vi "Array Max & Min JSON.vi"(7 "JSON Array":refnum<class "JSON Array.lvclass">, 11 "error in (no error)":errorcluster) -> (4 "max value":refnum<class "JSON Null.lvclass">, 6 "max index":i32, 8 "min value":refnum<class "JSON Null.lvclass">, 10 "min index":i32, 15 "error out":errorcluster)   [LabVIEW 2015, in "LVJSON.lvlib" / "JSON Array.lvclass"]
doc: "Finds the maximum value and minimum value of the elements in a JSON Array. The elements must all be the same literal type."
uses:
  JSON Array.lvclass
  JSON Datatype/JSON Null.lvclass
  JSON String/Read value (String).vi
  JSON Helper/To More Specific Type (String).vi
  JSON Numeric/Read value (Numeric).vi
  JSON Helper/To More Specific Type (Numeric).vi
  JSON Helper/JSON Helper.lvclass
  JSON Basic Type/JSON Literal.lvclass
  JSON Numeric/JSON Numeric.lvclass
  JSON String/JSON String.lvclass
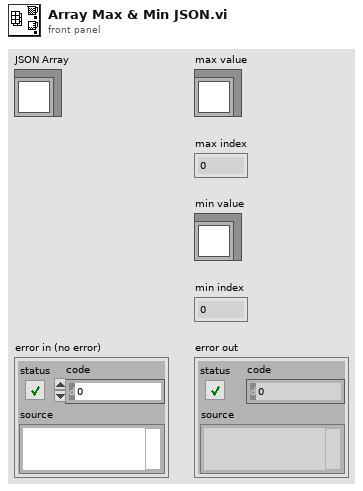
[diagram p1: front panel]
types:
  T1 = typedef "LVJSON.lvlib/JSON Types.ctl" = enum16{"String", "Numeric", "Boolean", "NULL", "Object", "Array"}
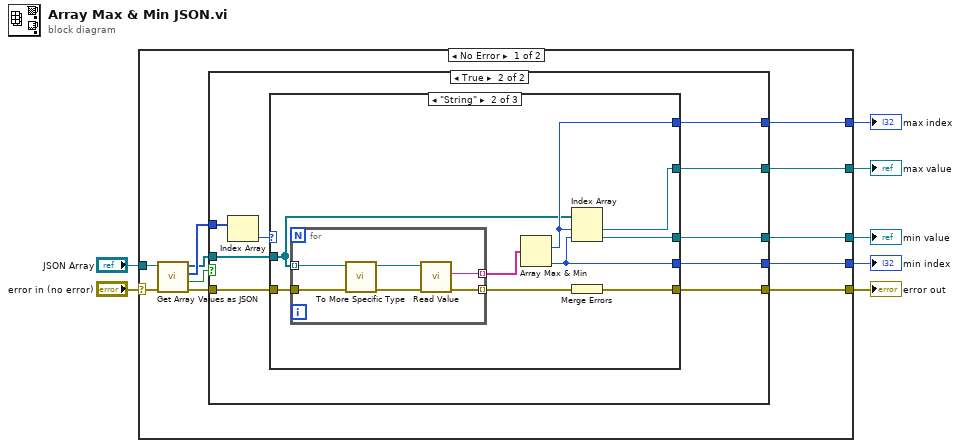
[diagram p0: block diagram]
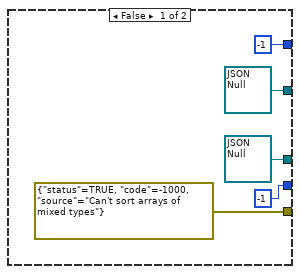
[diagram p2: hidden frame]
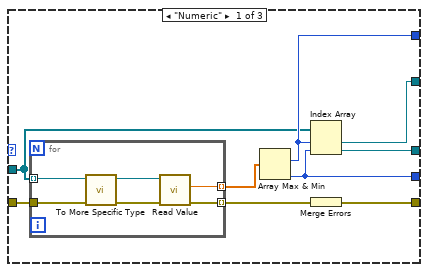
[diagram p3: hidden frame]
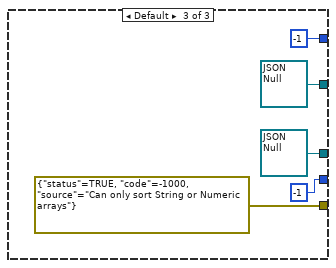
[diagram p4: hidden frame]
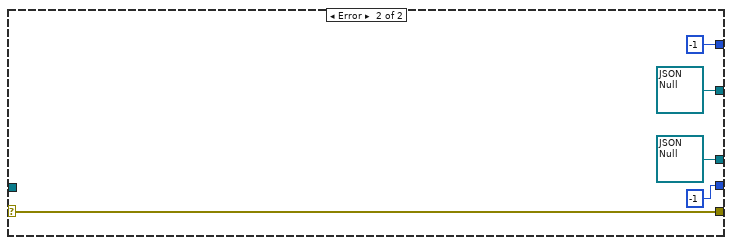
[diagram p5: hidden frame]
diagram:
  n1 = case shown="No Error" "error in (no error)" {
    selector: "error in (no error)" -> [w15 w72]
    tunnel: "JSON Array" -> [w13 _]
    tunnel: [w18 w72] -> w5
    tunnel: [w11 refnum<class "JSON Null.lvclass"> refnum ("JSON Datatype.lvclass")] -> w4
    tunnel: [w10 refnum<class "JSON Null.lvclass"> refnum ("JSON Datatype.lvclass")] -> w3
    tunnel: [w9 -1] -> w2
    tunnel: [w8 -1] -> w1
    frame No Error {
      n2 = call "Get Array Values as JSON.vi"("error in (no error)"=w15, "JSON Array in"=w13) -> ("error out"=w14:errorcluster, "single type?"=w16:bool, "types"=w17:T1[], "values"=w12:refnum<class "JSON Null.lvclass">[])  [unwired: 6 in]
      n3 = case shown="True" w16 {
        tunnel: w12 -> [_ w32]
        tunnel: w14 -> [_ w31]
        tunnel: [errorcluster {"status"=TRUE, "code"=-1000, "source"="Can't sort arrays of mixed types"} ("error IO") w30] -> w18
        tunnel: w17 -> [_ w29]
        tunnel: [refnum<class "JSON Null.lvclass"> refnum ("JSON Datatype.lvclass") w27] -> w11
        tunnel: [refnum<class "JSON Null.lvclass"> refnum ("JSON Datatype.lvclass") w26] -> w10
        tunnel: [-1 w25] -> w9
        tunnel: [-1 w24] -> w8
        frame False {
        }
        frame True {
          n4 = Index Array(array=w29) -> (element=w28:T1)  [unwired: 1 in]
          n5 = case shown="\"String\"" w28 {
            tunnel: w32 -> [w33 w48 _]
            tunnel: w31 -> [w41 w56 _]
            tunnel: [w38 w53 errorcluster {"status"=TRUE, "code"=-1000, "source"="Can only sort String or Numeric arrays"} ("error IO")] -> w30
            tunnel: [w37 w52 refnum<class "JSON Null.lvclass"> refnum ("JSON Datatype.lvclass")] -> w27
            tunnel: [w36 w51 refnum<class "JSON Null.lvclass"> refnum ("JSON Datatype.lvclass")] -> w26
            tunnel: [w35 w50 -1] -> w25
            tunnel: [w34 w49 -1] -> w24
            frame "Numeric" {
              n6 = for {
                tunnel: w33 -> [w47] mode=indexing
                tunnel: [w45] -> w40 mode=indexing
                tunnel: w41 -> [w44]
                tunnel: [w42] -> w39 mode=indexing
                n7 = call-poly "To More Specific Type.vi"("error in (no error)"=w44, "JSON Datatype in"=w47) -> ("error out"=w43:errorcluster, "JSON Numeric out"=w46:refnum<class "JSON Numeric.lvclass">)  [unwired: 8 in]
                n8 = call-poly "Read Value.vi"("error in (no error)"=w43, "JSON Numeric in"=w46) -> ("error out"=w42:errorcluster, "value"=w45:dbl)  [unwired: 8 in]
              }
              n9 = Array Max & Min(array=w40) -> (max index (indices)=w35:i32, min index (indices)=w34:i32)  [unwired: 2 out]
              n10 = Index Array(array=w33, index #1=w35, index #2=w34) -> (element #1=w37:refnum<class "JSON Null.lvclass">, element #2=w36:refnum<class "JSON Null.lvclass">)
              n11 = Merge Errors(w39) -> (w38:errorcluster)
            }
            frame "String" {
              n12 = for {
                tunnel: w48 -> [w62] mode=indexing
                tunnel: [w60] -> w55 mode=indexing
                tunnel: w56 -> [w59]
                tunnel: [w57] -> w54 mode=indexing
                n13 = call-poly "To More Specific Type.vi"("error in (no error)"=w59, "JSON Datatype in"=w62) -> ("error out"=w58:errorcluster, "JSON Datatype out"=w61:refnum<class "JSON String.lvclass">)  [unwired: 8 in]
                n14 = call-poly "Read Value.vi"("error in (no error)"=w58, "JSON String in"=w61) -> ("error out"=w57:errorcluster, "value"=w60:string)  [unwired: 8 in]
              }
              n15 = Array Max & Min(array=w55) -> (max index (indices)=w50:i32, min index (indices)=w49:i32)  [unwired: 2 out]
              n16 = Index Array(array=w48, index #1=w50, index #2=w49) -> (element #1=w52:refnum<class "JSON Null.lvclass">, element #2=w51:refnum<class "JSON Null.lvclass">)
              n17 = Merge Errors(w54) -> (w53:errorcluster)
            }
            frame Default {
            }
          }
        }
      }
    }
    frame Error {
    }
  }
  "error out" <- w5
  "max value" <- w4
  "min value" <- w3
  "max index" <- w2
  "min index" <- w1
